vi "VerifyNonNI_Instruments.vi"(5 "Instrument Types In":string[](array[string])) -> (2 "Instrument Types Out":string[](array[string]))   [LabVIEW 2021, in "Converter.lvlib"]
uses:
  Converter.lvlib
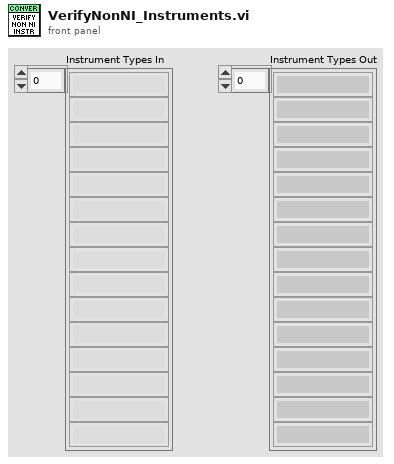
[diagram p1: front panel]
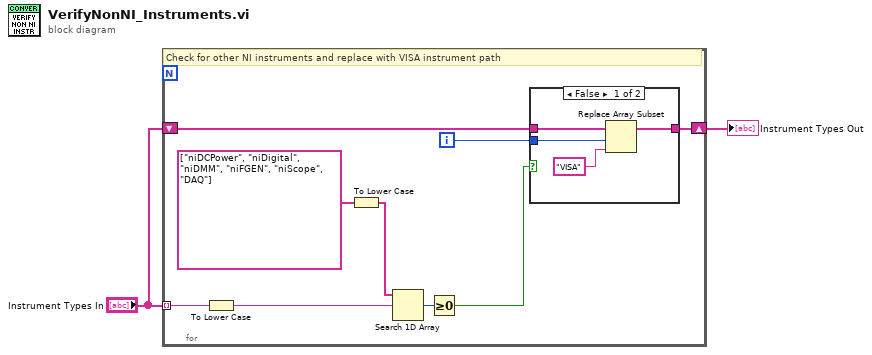
[diagram p0: block diagram]
diagram:
  n1 = for {
    tunnel: "Instrument Types In" -> [w10] mode=indexing
    shift-right: [w7] -> w1
    shift-left: "Instrument Types In" -> [w8]
    i -> [w6]
    # "Check for other NI instruments and replace with VISA instrument path"
    n2 = To Lower Case(string=w10) -> (all lower case string=w3:string)
    n3 = To Lower Case(string=string[] ["niDCPower", "niDigital", "niDMM", "niFGEN", "niScope", "DAQ"] ("regular expression")) -> (all lower case string=w5:string[])
    n4 = Search 1D Array(1D array=w5, element=w3) -> (index of element=w9:i32)  [unwired: 1 in]
    n5 = Greater Or Equal To 0?(x=w9) -> (x >= 0?=w4:bool)
    n6 = case shown="False" w4 {
      tunnel: w8 -> [w15 w16]
      tunnel: [w14 w16] -> w7
      tunnel: w6 -> [w13 _]
      frame False {
        n7 = Replace Array Subset(array=w15, new element="VISA" ("new element/subarray"), index=w13) -> (w14:string[])
      }
      frame True {
      }
    }
  }
  "Instrument Types Out" <- w1
